vi "HTTP-POSTRequest.vi"(6 "ResponseCode":string="201", 8 "error in (no error)":errorcluster, 9 "Buffer":string, 10 "Request":string, 11 "ByteGSWebAPI-V0 in":refnum<class "ByteGSWebAPI-V0.lvclass">) -> (0 "error out":errorcluster, 1 "Headers":string, 2 "Body":string, 3 "ByteGSWebAPI-V0 out":refnum<class "ByteGSWebAPI-V0.lvclass">)   [LabVIEW 2019, in "ByteGSWebAPI.lvlib" / "ByteGSWebAPI-V0.lvclass"]
doc: "Effettua una richiesta di Post al server come:\nSERVER/api/bytegs/RICHIESTA/"
uses:
  ByteGSWebAPI-V0.lvclass
  ByteGSWebAPI-V0.lvclass/ByteGSWebAPI-V0.ctl
  <vilib>/httpClient/POSTBuffer.vi
  <vilib>/httpClient/LabVIEWHTTPClient.lvlib
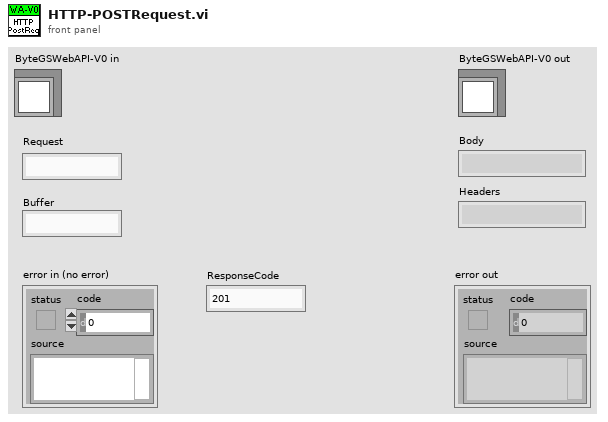
[diagram p1: front panel]
types:
  T1 = typedef "LabVIEWHTTPClient.lvlib/ClientHandle.ctl" = refnum<k1>
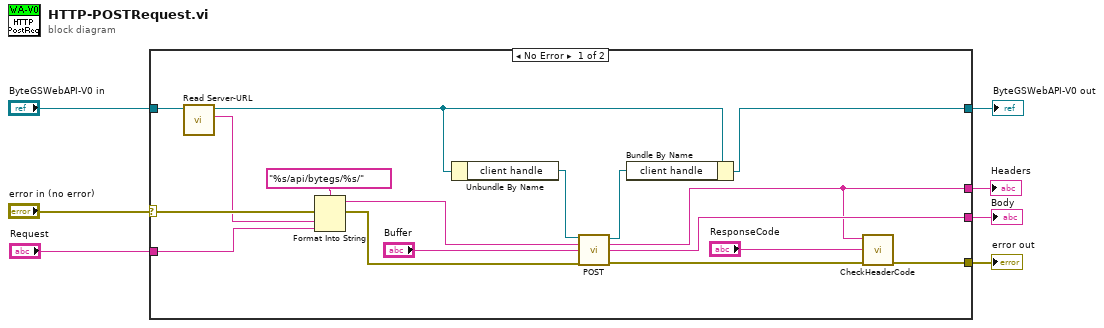
[diagram p0: block diagram]
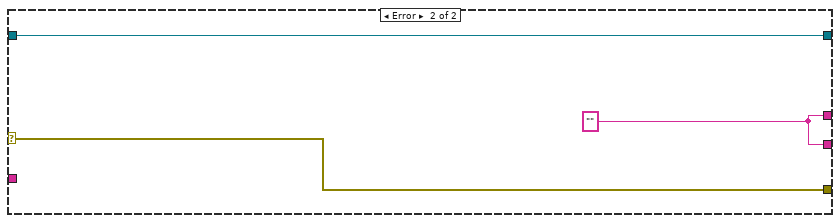
[diagram p2: hidden frame]
diagram:
  n1 = case shown="No Error" "error in (no error)" {
    selector: "error in (no error)" -> [w22 w27]
    tunnel: [w10 w27] -> w6
    tunnel: [w13 w26] -> w4
    tunnel: "ByteGSWebAPI-V0 in" -> [w24 w26]
    tunnel: "Request" -> [w21 _]
    tunnel: [w8 w25] -> w2
    tunnel: [w12 w25] -> w1
    frame No Error {
      n2 = call-dynamic "Read Server-URL.vi"("ByteGSWebAPI-V0 in"=w24) -> ("Server-URL"=w20:string, "ByteGSWebAPI-V0 out"=w14:refnum<class "ByteGSWebAPI-V0.lvclass">)  [unwired: 8 in, 1 out]
      n3 = Format Into String(format string="%s/api/bytegs/%s/" ("url"), error in=w22, w20, w21) -> (resulting string=w18:string, error out=w19:errorcluster)  [unwired: 1 in]
      n4 = Unbundle By Name(w14) -> ("client handle"=w16:T1)
      n5 = call-poly <vilib>:"POST.vi"("client handle"=w16, "url"=w18, "buffer"="Buffer", "error in (no error)"=w19) -> ("client handle out"=w15:T1, "headers"=w8:string, "body"=w12:string, "error out"=w11:errorcluster)  [unwired: 8 in]
      n6 = Bundle By Name(cluster=w14, "client handle"=w15) -> (w13:refnum<class "ByteGSWebAPI-V0.lvclass">)
      n7 = call "CheckHeaderCode.vi"("error in"=w11, "Code"="ResponseCode", "Headers"=w8) -> ("error out"=w10:errorcluster)  [unwired: 8 in]
    }
    frame Error {
      w25 = "" ("headers")
    }
  }
  "error out" <- w6
  "ByteGSWebAPI-V0 out" <- w4
  "Headers" <- w2
  "Body" <- w1
